vi "Switch_off_Temp_Rise_meas_during_SG_tupe_rapture.vi"(0 "SI100_ReactorTemperatureRise.lvclass":refnum<class "SI100.lvclass">, 1 "GM61 R1":bool, 2 "GM61 R2":bool, 3 "GM61 R3":bool, 4 "GM61 R4":bool, 5 "error in":errorcluster, 6 "Temp.-Rise 2nd Max R1":dbl format="%#_13g", 7 "Temp.-Rise 2nd Max R3":dbl format="%#_13g", 8 "Temp.-Rise 2nd Max R2":dbl format="%#_13g", 9 "Temp.-Rise 2nd Max R4":dbl format="%#_13g") -> (14 "SI100_ReactorTemperatureRise.lvclass out":refnum<class "SI100.lvclass">, 15 "R1":T4, 16 "R2":T3, 17 "R3":T2, 18 "R4":T1, 19 "error IO":errorcluster)   [LabVIEW 2022 SP3, in "SI100.lvclass"]
uses:
  SI100.lvclass
  SI100.lvclass/SI100.ctl
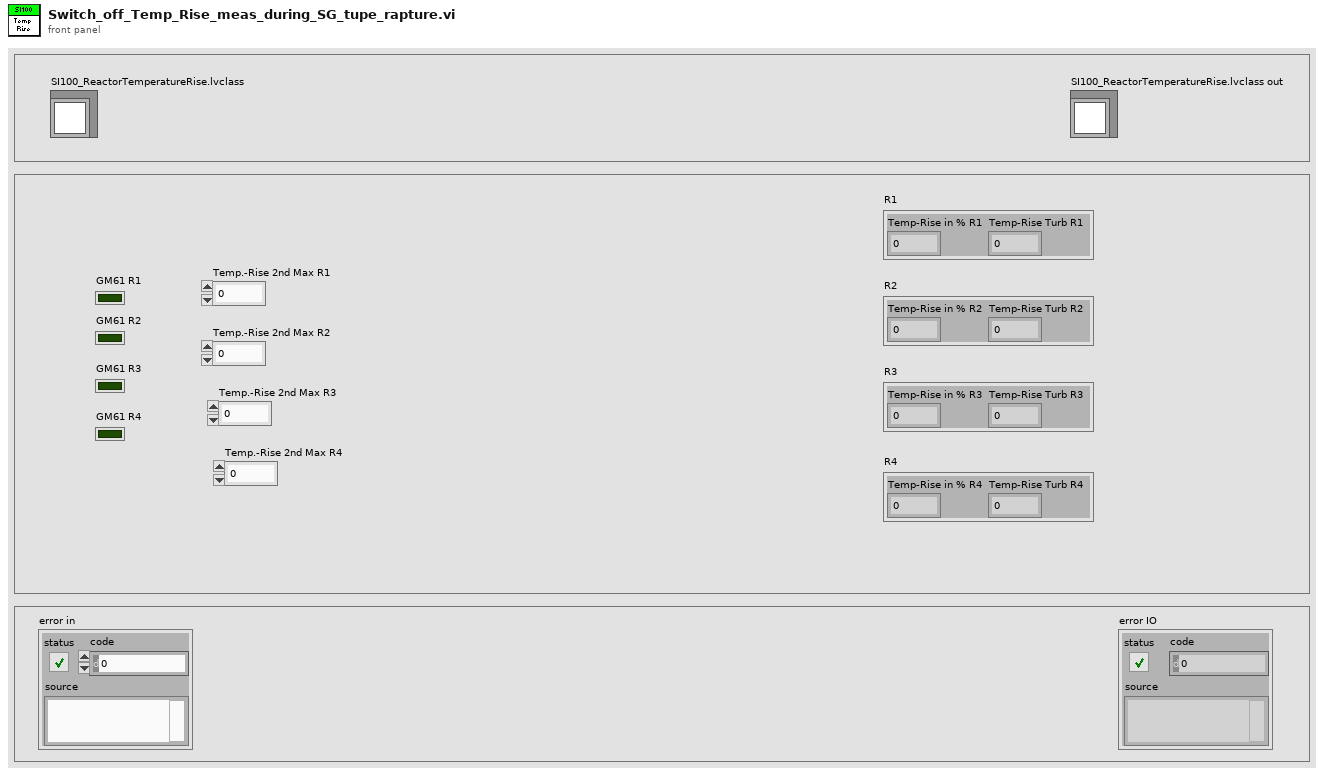
[diagram p1: front panel]
types:
  T1 = cluster{"Temp-Rise in % R4":dbl, "Temp-Rise Turb R4":dbl}
  T2 = cluster{"Temp-Rise in % R3":dbl, "Temp-Rise Turb R3":dbl}
  T3 = cluster{"Temp-Rise in % R2":dbl, "Temp-Rise Turb R2":dbl}
  T4 = cluster{"Temp-Rise in % R1":dbl, "Temp-Rise Turb R1":dbl}
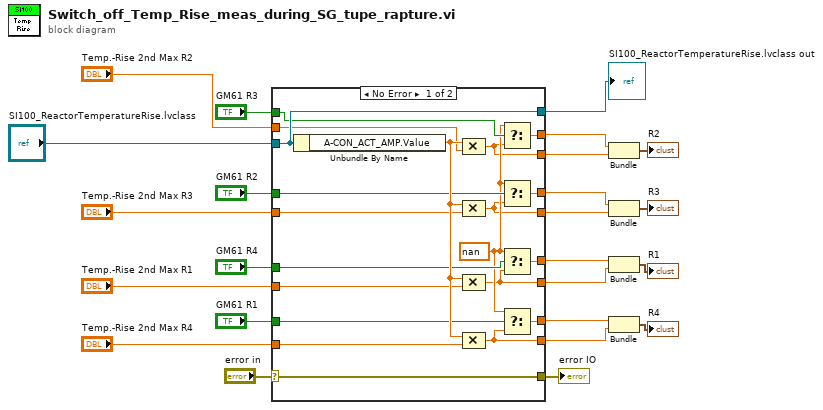
[diagram p0: block diagram]
diagram:
  n1 = case shown="No Error" "error in" {
    selector: "error in" -> [w29 w45]
    tunnel: "GM61 R1" -> [w42 _]
    tunnel: "GM61 R2" -> [w41 _]
    tunnel: "GM61 R3" -> [w40 _]
    tunnel: "GM61 R4" -> [w39 _]
    tunnel: "SI100_ReactorTemperatureRise.lvclass" -> [w43 w46]
    tunnel: [w43 w46] -> w19
    tunnel: [w37 _] -> w10
    tunnel: [w36 _] -> w12
    tunnel: [w35 _] -> w14
    tunnel: [w34 _] -> w16
    tunnel: [w33 _] -> w9
    tunnel: [w32 _] -> w11
    tunnel: [w31 _] -> w13
    tunnel: [w30 _] -> w15
    tunnel: [w29 w45] -> w17
    tunnel: "Temp.-Rise 2nd Max R1" -> [w28 _]
    tunnel: "Temp.-Rise 2nd Max R2" -> [w27 _]
    tunnel: "Temp.-Rise 2nd Max R3" -> [w26 _]
    tunnel: "Temp.-Rise 2nd Max R4" -> [w25 _]
    frame No Error {
      w38 = nan
      n2 = Unbundle By Name(w43) -> ("A-CON_ACT_AMP.Value"=w44:dbl)
      n3 = Compound Arithmetic op=MULTIPLY(w44, w27) -> (w31:dbl)
      n4 = Compound Arithmetic op=MULTIPLY(w44, w26) -> (w32:dbl)
      n5 = Compound Arithmetic op=MULTIPLY(w44, w28) -> (w30:dbl)
      n6 = Compound Arithmetic op=MULTIPLY(w44, w25) -> (w33:dbl)
      n7 = Select(t=w38, s=w40, f=w31) -> (s? t:f=w35:dbl)
      n8 = Select(t=w38, s=w41, f=w32) -> (s? t:f=w36:dbl)
      n9 = Select(t=w38, s=w39, f=w30) -> (s? t:f=w34:dbl)
      n10 = Select(t=w38, s=w42, f=w33) -> (s? t:f=w37:dbl)
    }
    frame Error {
    }
  }
  "SI100_ReactorTemperatureRise.lvclass out" <- w19
  "error IO" <- w17
  n11 = Bundle(w14, w13) -> (→"R2":cluster{dbl, dbl})  [unwired: 1 in]
  n12 = Bundle(w12, w11) -> (→"R3":cluster{dbl, dbl})  [unwired: 1 in]
  n13 = Bundle(w16, w15) -> (→"R1":cluster{dbl, dbl})  [unwired: 1 in]
  n14 = Bundle(w10, w9) -> (→"R4":cluster{dbl, dbl})  [unwired: 1 in]
